vi "set_idn.vi"(0 "HGF_DeviceBase":refnum<class "HGF_DeviceBase.lvclass">, 1 "driverRevision":string="unknown", 2 "firmwareRevision":string="unknown", 3 "vendor":string="unknown", 4 "model":string="unknown", 5 "error in (no error)":errorcluster) -> (14 "dup HGF_DeviceBase":refnum<class "HGF_DeviceBase.lvclass">, 19 "error out":errorcluster)   [LabVIEW 2014, in "HGF_DeviceBaseClasses.lvlib" / "HGF_DeviceBase.lvclass"]
doc: "write instrument driver revision, firmware revision, vendor, model, etc."
uses:
  HGF_DeviceBase.lvclass
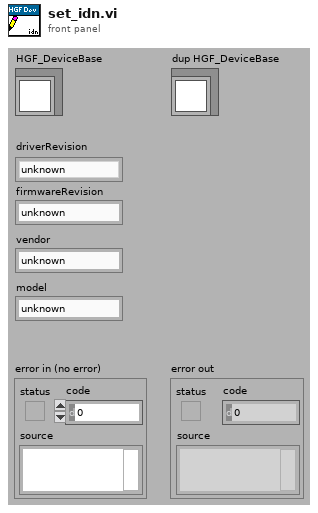
[diagram p1: front panel]
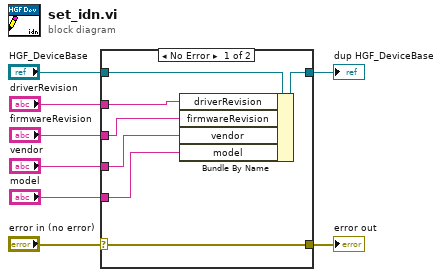
[diagram p0: block diagram]
diagram:
  n1 = case shown="No Error" "error in (no error)" {
    selector: "error in (no error)" -> [w15 w16]
    tunnel: [w15 w16] -> w7
    tunnel: [w13 w17] -> w5
    tunnel: "HGF_DeviceBase" -> [w14 w17]
    tunnel: "driverRevision" -> [w12 _]
    tunnel: "firmwareRevision" -> [w11 _]
    tunnel: "vendor" -> [w10 _]
    tunnel: "model" -> [w9 _]
    frame No Error {
      n2 = Bundle By Name(cluster=w14, "driverRevision"=w12, "firmwareRevision"=w11, "vendor"=w10, "model"=w9) -> (w13:refnum<class "HGF_DeviceBase.lvclass">)
    }
    frame Error {
    }
  }
  "error out" <- w7
  "dup HGF_DeviceBase" <- w5
